vi "Calculate Index Array.vi"(8 "error in (no error)":errorcluster, 10 "3D Pie Datatype.lvclass in":refnum<class "3D Pie Datatype.lvclass">, 11 "Plot Representation In":T1) -> (0 "error out":errorcluster, 2 "3D Pie Datatype.lvclass out":refnum<class "3D Pie Datatype.lvclass">, 3 "Plot Representation Out":T1)   [LabVIEW 2017, in "3D Pie Datatype.lvclass"]
uses:
  <vilib>/Math Plots/3D Math Plots/3D Pie/3D Pie Datatype/3D Pie Datatype.lvclass
  <vilib>/Math Plots/3D Math Plots/3D Plot/3D Plot/Typedef/Plot Representation.ctl
  <vilib>/Math Plots/3D Math Plots/3D Plot/3D Plot/Typedef/Range Clusters.ctl
  <vilib>/Math Plots/3D Math Plots/3D Plot/3D Plot/Typedef/Mesh Data.ctl
  <vilib>/Math Plots/3D Math Plots/3D Plot/3D Plot/3D Plot.lvclass
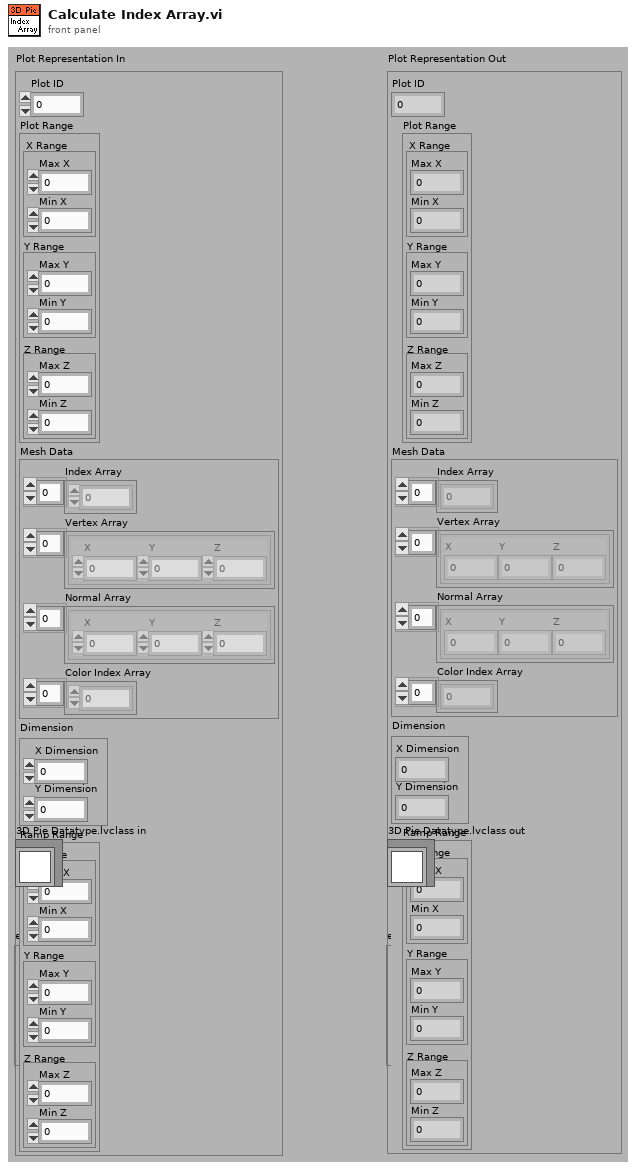
[diagram p1: front panel]
types:
  T1 = typedef "3D Plot.lvclass/Plot Representation.ctl" = cluster{"Plot ID":i32, "Plot Range":T2, "Mesh Data":T3, "Dimension":cluster{"X Dimension":i32, "Y Dimension":i32}, "Ramp Range":T2}
  T2 = typedef "3D Plot.lvclass/Range Clusters.ctl" = cluster{"X Range":cluster{"Max X":sgl, "Min X":sgl}, "Y Range":cluster{"Max Y":sgl, "Min Y":sgl}, "Z Range":cluster{"Max Z":sgl, "Min Z":sgl}}
  T3 = typedef "3D Plot.lvclass/Mesh Data.ctl" = cluster{"Index Array":u32[], "Vertex Array":cluster{"X":sgl, "Y":sgl, "Z":sgl}[], "Normal Array":cluster{"X":sgl, "Y":sgl, "Z":sgl}[], "Color Index Array":i32[]}
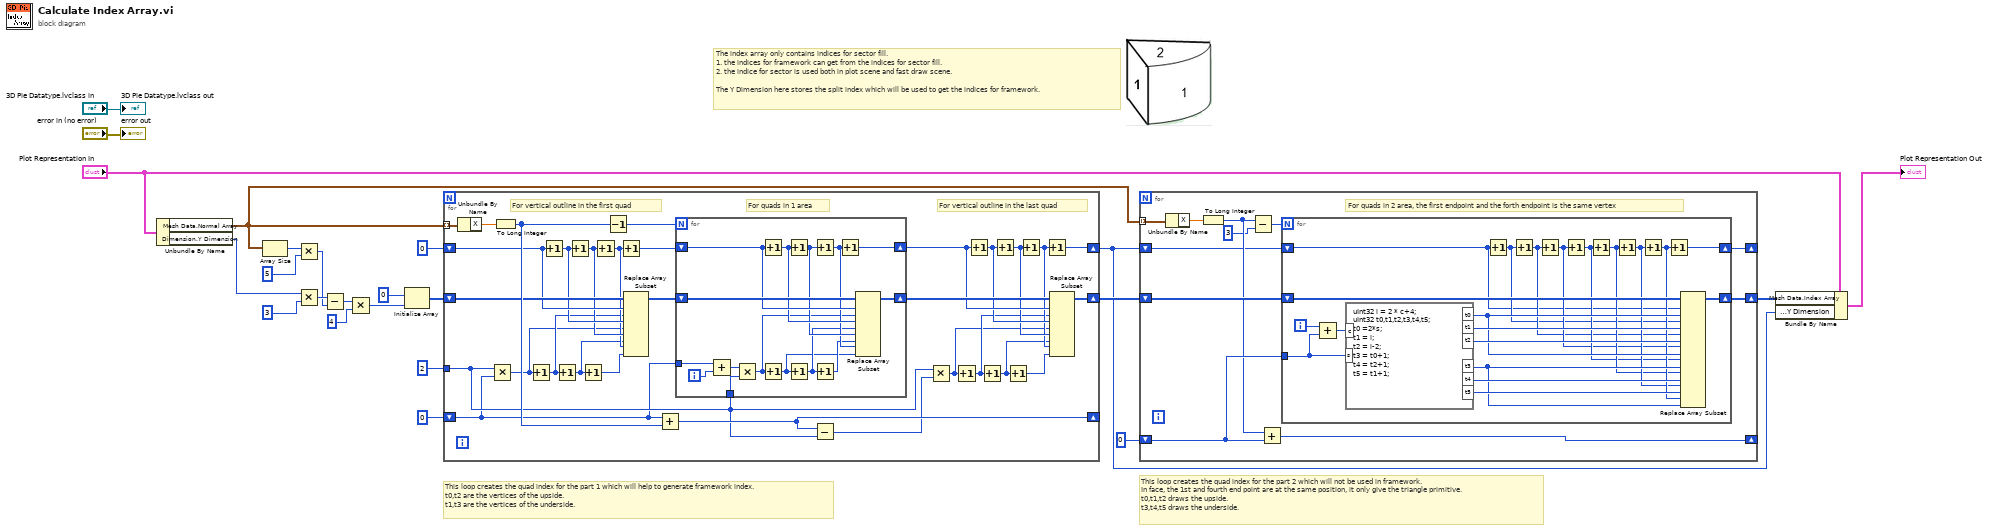
[diagram p0: block diagram]
diagram:
  # "This loop creates the quad index for the part 2 which will not be used in framework.\nIn face, the 1st and fourth end point are at the same position, it only give the triangle primitive.\nt0,t1,t2 draws the upside.\nt3,t4,t5 draws the underside."
  # "This loop creates the quad index for the part 1 which will help to generate framework index.\nt0,t2 are the vertices of the upside.\nt1,t3 are the vertices of the underside."
  # "The index array only contains indices for sector fill.\n1. the indices for framework can get from the indices for sector fill.\n2. the indice for sector is used both in plot scene and fast draw scene.\n\nThe Y Dimension here stores the split index which will be used to get the indices for framework."
  n1 = Unbundle By Name("Plot Representation In") -> ("Mesh Data.Normal Array"=w14:cluster{"X":sgl, "Y":sgl, "Z":sgl}[], "Dimension.Y Dimension"=w12:i32)
  n2 = Array Size(array=w14) -> (size(s)=w13:i32)
  n3 = Multiply(x=w13, y=5) -> (x*y=w8:i32)
  n4 = Multiply(x=w12, y=3) -> (x*y=w9:i32)
  n5 = Subtract(x=w9, y=w8) -> (x-y=w6:i32)
  n6 = Multiply(x=w6, y=4 ("x")) -> (x*y=w3:i32)
  n7 = Initialize Array(u32 0 ("element"), w3) -> (w7:u32[])
  n8 = for {
    tunnel: w14 -> [w52] mode=indexing
    shift-right: [w40] -> w16
    shift-left: w7 -> [w43]
    shift-right: [w49] -> _
    shift-left: u32 0 -> [w44]
    shift-right: [w47] -> w4
    shift-left: 0 -> [w35]
    tunnel: u32 2 ("y") -> [w45]
    # "For vertical outline in the last quad"
    # "For vertical outline in the first quad"
    # "For quads in 1 area"
    n9 = Unbundle By Name(w52) -> ("X"=w50:sgl)
    n10 = Multiply(x=w45, y=w44) -> (x*y=w30:u32)
    n11 = To Long Integer(number=w50) -> (32bit integer=w51:i32)
    n12 = Increment(x=w30) -> (x+1=w31:u32)
    n13 = Increment(x=w35) -> (x+1=w34:i32)
    n14 = Increment(x=w31) -> (x+1=w29:u32)
    n15 = Increment(x=w34) -> (x+1=w33:i32)
    n16 = Increment(x=w29) -> (x+1=w28:u32)
    n17 = Increment(x=w33) -> (x+1=w32:i32)
    n18 = Decrement(x=w51) -> (x-1=w53:i32)
    n19 = Increment(x=w32) -> (x+1=w48:i32)
    n20 = Replace Array Subset(array=w43, new element #1=w31, index #1=w35, new element #2=w30, index #2=w34, new element #3=w29, index #3=w33, new element #4=w28, index #4=w32) -> (w42:u32[])
    n21 = Add(x=w44, y=w51) -> (x+y=w49:u32)
    n22 = for {
      N: w53 -> [_]
      shift-right: [w62] -> w41
      shift-left: w42 -> [w63]
      tunnel: w44 -> [w67]
      shift-right: [w66] -> w39
      shift-left: w48 -> [w61]
      tunnel: w45 -> [w64]
      i -> [w68]
      n23 = Add(x=w67, y=w68) -> (x+y=w65:u32)
      n24 = Multiply(x=w65, y=w64) -> (x*y=w57:u32)
      n25 = Increment(x=w61) -> (x+1=w60:i32)
      n26 = Increment(x=w57) -> (x+1=w54:u32)
      n27 = Increment(x=w60) -> (x+1=w59:i32)
      n28 = Increment(x=w54) -> (x+1=w56:u32)
      n29 = Increment(x=w59) -> (x+1=w58:i32)
      n30 = Increment(x=w56) -> (x+1=w55:u32)
      n31 = Increment(x=w58) -> (x+1=w66:i32)
      n32 = Replace Array Subset(array=w63, new element #1=w57, index #1=w61, new element #2=w56, index #2=w60, new element #3=w55, index #3=w59, new element #4=w54, index #4=w58) -> (w62:u32[])
    }
    n33 = Subtract(x=w49, y=w45) -> (x-y=w46:u32)
    n34 = Multiply(x=w45, y=w46) -> (x*y=w26:u32)
    n35 = Increment(x=w26) -> (x+1=w27:u32)
    n36 = Increment(x=w39) -> (x+1=w38:i32)
    n37 = Increment(x=w27) -> (x+1=w25:u32)
    n38 = Increment(x=w38) -> (x+1=w37:i32)
    n39 = Increment(x=w25) -> (x+1=w24:u32)
    n40 = Increment(x=w37) -> (x+1=w36:i32)
    n41 = Increment(x=w36) -> (x+1=w47:i32)
    n42 = Replace Array Subset(array=w41, new element #1=w27, index #1=w39, new element #2=w26, index #2=w38, new element #3=w25, index #3=w37, new element #4=w24, index #4=w36) -> (w40:u32[])
  }
  n43 = for {
    tunnel: w14 -> [w73] mode=indexing
    shift-right: [w75] -> w17
    shift-left: w16 -> [w79]
    shift-right: [w78] -> _
    shift-left: 0 -> [w77]
    shift-right: [w69] -> _
    shift-left: w4 -> [w70]
    # "For quads in 2 area, the first endpoint and the forth endpoint is the same vertex"
    n44 = Unbundle By Name(w73) -> ("X"=w74:sgl)
    n45 = To Long Integer(number=w74) -> (32bit integer=w72:i32)
    n46 = Subtract(x=w72, y=3 ("x")) -> (x-y=w76:i32)
    n47 = Add(x=w72, y=w77) -> (x+y=w78:i32)
    n48 = for {
      N: w76 -> [_]
      shift-right: [w95] -> w75
      shift-left: w79 -> [w88]
      tunnel: w77 -> [w97]
      shift-right: [w96] -> w69
      shift-left: w70 -> [w80]
      i -> [w99]
      n49 = Add(x=w99, y=w97) -> (x+y=w98:i32)
      n50 = formula code="uInt32 i = 2 * c+4; \nuInt32 t0,t1,t2,t3,t4,t5;\nt0 =2*s; \nt1 = i; \nt2 = i-2;\nt3 = t0+1;\nt4 = t2+1;\nt5 = t1+1;"("c"=w98, "s"=w97) -> ("t0"=w92:u32, "t1"=w94:u32, "t2"=w93:u32, "t3"=w89:u32, "t4"=w91:u32, "t5"=w90:u32)
      n51 = Increment(x=w80) -> (x+1=w81:i32)
      n52 = Increment(x=w81) -> (x+1=w82:i32)
      n53 = Increment(x=w82) -> (x+1=w83:i32)
      n54 = Increment(x=w83) -> (x+1=w84:i32)
      n55 = Increment(x=w84) -> (x+1=w85:i32)
      n56 = Increment(x=w85) -> (x+1=w86:i32)
      n57 = Increment(x=w86) -> (x+1=w87:i32)
      n58 = Increment(x=w87) -> (x+1=w96:i32)
      n59 = Replace Array Subset(array=w88, new element #1=w92, index #1=w80, new element #2=w94, index #2=w81, new element #3=w93, index #3=w82, new element #4=w92, index #4=w83, new element #5=w89, index #5=w84, new element #6=w91, index #6=w85, new element #7=w90, index #7=w86, new element #8=w89, index #8=w87) -> (w95:u32[])
    }
  }
  n60 = Bundle By Name(cluster="Plot Representation In", "Mesh Data.Index Array"=w17, "Dimension.Y Dimension"=w4) -> (→"Plot Representation Out":T1)
  "error out" <- "error in (no error)"
  "3D Pie Datatype.lvclass out" <- "3D Pie Datatype.lvclass in"
